vi "Status.vi"(8 "error in (no error)":errorcluster, 11 "Serial Controller in":refnum<class "Serial Controller.lvclass">) -> (0 "error out":errorcluster, 2 "Firmware Version":u16, 3 "Serial Controller out":refnum<class "Serial Controller.lvclass">)   [LabVIEW 2011, in "Serial Controller.lvclass"]
uses:
  Serial Controller.lvclass
  Serial Controller.lvclass/Serial Controller.ctl
panel:
  out "StepDiv":u16
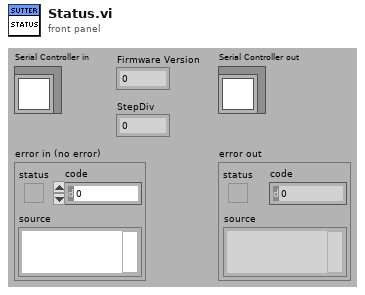
[diagram p1: front panel]
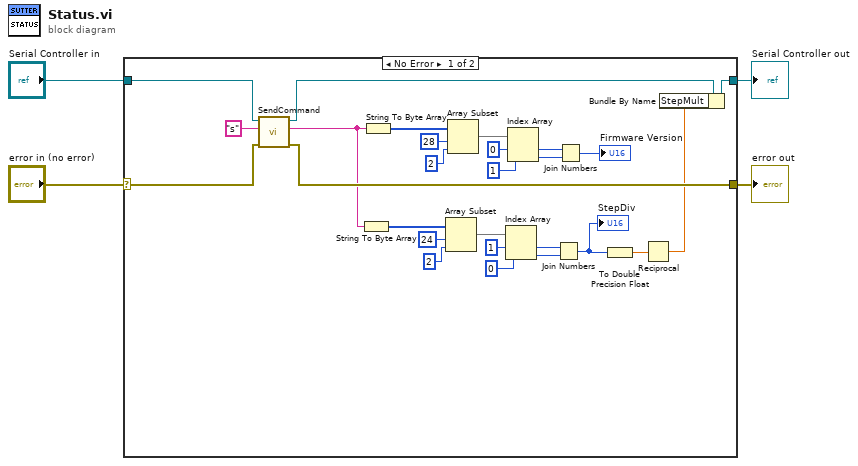
[diagram p0: block diagram]
diagram:
  n1 = case shown="No Error" "error in (no error)" {
    selector: "error in (no error)" -> [w21 w33]
    tunnel: [w20 w33] -> w3
    tunnel: [w5 w32] -> w1
    tunnel: "Serial Controller in" -> [w22 w32]
    frame No Error {
      n2 = call-dynamic "SendCommand.vi"("error in (no error)"=w21, "command"="s", "Serial Controller in"=w22) -> ("error out"=w20:errorcluster, "Returned"=w10:string, "Serial Controller out"=w6:refnum<class "Serial Controller.lvclass">)  [unwired: 6 in]
      n3 = String To Byte Array(string=w10) -> (unsigned byte array=w18:u8[])
      n4 = String To Byte Array(string=w10) -> (unsigned byte array=w31:u8[])
      n5 = Array Subset(array=w18, index=24, length=2) -> (w15:u8[])
      n6 = Array Subset(array=w31, index=28, length=2) -> (w28:u8[])
      n7 = Index Array(array=w15, index #1=1 ("index"), index #2=0 ("index")) -> (element #1=w12:u8, element #2=w11:u8)
      n8 = Index Array(array=w28, index #1=0 ("index"), index #2=1 ("index")) -> (element #1=w25:u8, element #2=w24:u8)
      n9 = Join Numbers(hi=w12, lo=w11) -> ((hi.lo)=w8:u16)
      "StepDiv" <- w8
      n10 = Join Numbers(hi=w25, lo=w24) -> ((hi.lo)=→"Firmware Version":u16)
      n11 = To Double Precision Float(number=w8) -> (double precision float=w7:dbl)
      n12 = Reciprocal(x=w7) -> (1/x=w9:dbl)
      n13 = Bundle By Name(cluster=w6, "StepMult"=w9) -> (w5:refnum<class "Serial Controller.lvclass">)
    }
    frame Error {
    }
  }
  "error out" <- w3
  "Serial Controller out" <- w1
